vi "map.vi"(7 "value":sgl, 8 "newMax":i32, 9 "newMin":i32, 10 "oldMax":sgl, 11 "oldMin":sgl) -> (2 "newValue":i32)   [LabVIEW 2016]
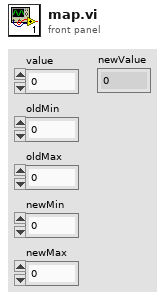
[diagram p1: front panel]
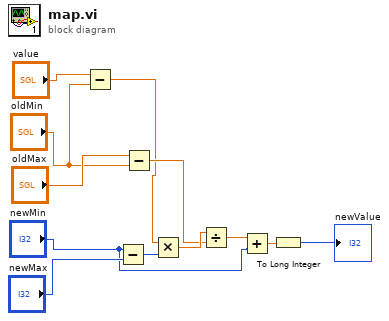
[diagram p0: block diagram]
diagram:
  n1 = Subtract(x="value", y="oldMin") -> (x-y=w5:sgl)
  n2 = Subtract(x="newMin", y="newMax") -> (x-y=w10:i32)
  n3 = Subtract(x="oldMax", y="oldMin") -> (x-y=w8:sgl)
  n4 = Multiply(x=w5, y=w10) -> (x*y=w9:sgl)
  n5 = Divide(x=w9, y=w8) -> (x/y=w4:sgl)
  n6 = Add(x=w4, y="newMin") -> (x+y=w2:sgl)
  n7 = To Long Integer(number=w2) -> (32bit integer=→"newValue":i32)
